vi "String to XYZ.vi"(0 "Input string":string) -> (14 "X":dbl, 15 "Y":dbl, 16 "Z":dbl, 17 "X Has Value?":bool, 18 "Y Has Value?":bool, 19 "Z Has Value?":bool)   [LabVIEW 2011]
uses:
  <vilib>/regexp/Match Regular Expression.xnode
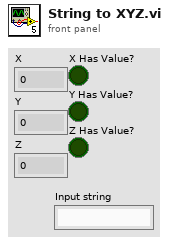
[diagram p1: front panel]
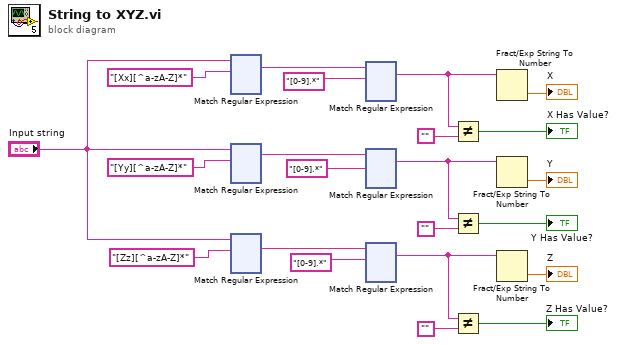
[diagram p0: block diagram]
diagram:
  n1 = xnode "Match Regular Expression"("input string"="Input string", "regular expression"="[Xx][^a-zA-Z]*") -> ("whole match"=w17:string)  [unwired: 4 in, 4 out]
  n2 = xnode "Match Regular Expression"("input string"="Input string", "regular expression"="[Yy][^a-zA-Z]*") -> ("whole match"=w13:string)  [unwired: 4 in, 4 out]
  n3 = xnode "Match Regular Expression"("input string"="Input string", "regular expression"="[Zz][^a-zA-Z]*") -> ("whole match"=w14:string)  [unwired: 4 in, 4 out]
  n4 = xnode "Match Regular Expression"("input string"=w17, "regular expression"="[0-9].*") -> ("whole match"=w11:string)  [unwired: 4 in, 4 out]
  n5 = xnode "Match Regular Expression"("input string"=w13, "regular expression"="[0-9].*") -> ("whole match"=w9:string)  [unwired: 4 in, 4 out]
  n6 = xnode "Match Regular Expression"("input string"=w14, "regular expression"="[0-9].*") -> ("whole match"=w8:string)  [unwired: 4 in, 4 out]
  n7 = Not Equal?(x=w11, y="") -> (x != y?=→"X Has Value?":bool)
  n8 = Not Equal?(x=w9, y="") -> (x != y?=→"Y Has Value?":bool)
  n9 = Not Equal?(x=w8, y="") -> (x != y?=→"Z Has Value?":bool)
  n10 = Fract/Exp String To Number(string=w11) -> (number=→"X":dbl)  [unwired: 3 in, 1 out]
  n11 = Fract/Exp String To Number(string=w9) -> (number=→"Y":dbl)  [unwired: 3 in, 1 out]
  n12 = Fract/Exp String To Number(string=w8) -> (number=→"Z":dbl)  [unwired: 3 in, 1 out]
